vi "Initialize Attributes.vi"(8 "error in (no error)":errorcluster, 10 "Attribute Data":variant, 11 "CS++RTMessageLogger in":refnum<class "CS++RTMessageLogger.lvclass">) -> (0 "error out":errorcluster, 2 "Found?":bool, 3 "CS++RTMessageLogger out":refnum<class "CS++RTMessageLogger.lvclass">)   [LabVIEW 2015, in "CS++RTClasses.lvlib" / "CS++RTMessageLogger.lvclass"]
doc: "Initialize object attribute.\n\nUnique resources should be allocated elsewhere!"
uses:
  CS++RTMessageLogger.lvclass
  CS++RTMessageLogger.lvclass/CS++RTMessageLogger.ctl
  CSPP_Core/Classes/CS++BaseClasses/MessageLogger/CS++MessageLogger.lvclass
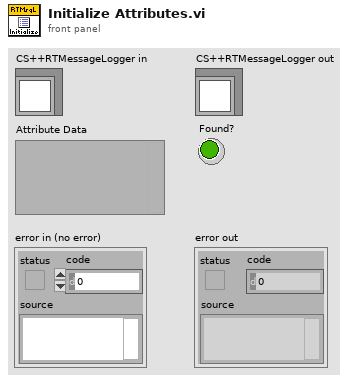
[diagram p1: front panel]
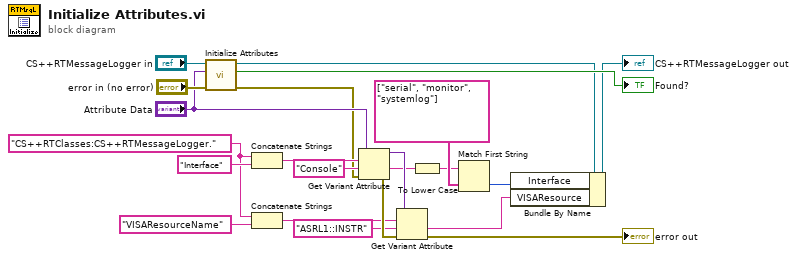
[diagram p0: block diagram]
diagram:
  w12 = "CS++RTClasses:CS++RTMessageLogger."
  n1 = call-parent "Initialize Attributes.vi"("error in (no error)"="error in (no error)", "Attribute Data"="Attribute Data", "CS++Base in"="CS++RTMessageLogger in") -> ("error out"=w9:errorcluster, "Found?"=→"Found?":bool, "CS++Base out"=w7:refnum<class "CS++RTMessageLogger.lvclass">)  [unwired: 6 in]
  n2 = Concatenate Strings(w12, "Interface" ("string")) -> (w18:string)
  n3 = Concatenate Strings(w12, "VISAResourceName" ("string")) -> (w11:string)
  n4 = Get Variant Attribute(Variant="Attribute Data", name=w18, default value (empty Variant)="Console" ("string"), error in=w9) -> (duplicate Variant=w14:variant, value=w5:string, error out=w15:errorcluster)  [unwired: 1 out]
  n5 = Get Variant Attribute(Variant=w14, name=w11, default value (empty Variant)="ASRL1::INSTR" ("string"), error in=w15) -> (value=w4:string, error out=→"error out":errorcluster)  [unwired: 2 out]
  n6 = To Lower Case(string=w5) -> (all lower case string=w2:string)
  n7 = Match First String(2:string[] ["serial", "monitor", "systemlog"], 3:w2) -> (0:w1:i32)  [unwired: 1 out]
  n8 = Bundle By Name(cluster=w7, "Interface"=w1, "VISAResource"=w4) -> (→"CS++RTMessageLogger out":refnum<class "CS++RTMessageLogger.lvclass">)
